vi "niRFUtil MEAS Mean (real wfm).vi"(7 "Waveform In":T1 {"y" min=0 max=127 format="%.2f"; "dx" format="%^.2e"; "x0" format="%^.2e"}) -> (8 "Mean":sgl format="%.2f")   [LabVIEW 2015, in "niRFUtil.lvlib"]
doc: "(c) Copyright 2006, National Instruments, Inc. This VI may not be duplicated, sold, or distributed without written consent from National Instruments."
uses:
  niRFUtil.lvlib
  Includes/niRFUtil INC Real Waveform.ctl
  Includes/niRFUtil INC Real Array.ctl
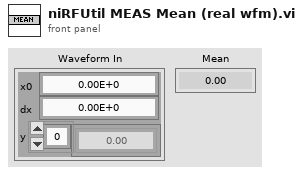
[diagram p1: front panel]
types:
  T1 = typedef "niRFUtil.lvlib/niRFUtil INC Real Waveform.ctl" = cluster{"x0":dbl, "dx":dbl, "y":T2}
  T2 = typedef "niRFUtil.lvlib/niRFUtil INC Real Array.ctl" = sgl[]
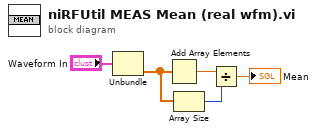
[diagram p0: block diagram]
diagram:
  n1 = Unbundle("Waveform In") -> ("y"=w4:T2)  [unwired: 2 out]
  n2 = Add Array Elements(numeric array=w4) -> (sum=w3:sgl)
  n3 = Array Size(array=w4) -> (size(s)=w2:i32)
  n4 = Divide(x=w3, y=w2) -> (x/y=→"Mean":sgl)
